vi "Test_for_6581.vi"() -> ()   [LabVIEW 2018]
uses:
  <vilib>/Platform/TimedLoop/XDataNode/timing_clust.ctl
  <vilib>/Platform/TimedLoop/XDataNode/nitl_modes.ctl
  <vilib>/Platform/TimedLoop/XDataNode/wakeup.ctl
  <vilib>/rvi/eio/common/nirviEmuTemplateMethod_errors.vi
  <vilib>/rvi/Emulation/niFpgaSctlEmulationGetInTimedLoop.vi
  <vilib>/rvi/Emulation/niFpgaEmulationReportErrorSimple.vi
  <vilib>/rvi/Emulation/niFpgaGetClockAttributes.vi
  <vilib>/rvi/Emulation/niFpgaCriticalErrorInLSC.vi
  <vilib>/eio/EIONode/EIONode.xnode
  <vilib>/Platform/TimedLoop/XDataNode/XDataNode.xnode
  <vilib>/Platform/TimedLoop/XDataNode/XDNodeRunTimeDep.lvlib
panel:
  in  "Internal Power Supply Voltage":u8(ring) items=["3.3 Volts", "2.5 Volts", "1.8 Volts"]
  in  "Supply Select":u8(ring) items=["Local", "External"]
  in  "Devider Frequency 160/(x*2), x>0":u8=1 min=1
  in  "Constant(F) / Frequency(T)":bool
  in  "IO Module\\DDCB_PFI3_Write":bool
  in  "IO Module\\DDCB_PFI2_Write":bool
  in  "IO Module\\DDCB_PFI1_Write":bool
  in  "IO Module\\DDCB_DIO23_Write":bool
  in  "IO Module\\DDCB_DIO22_Write":bool
  in  "IO Module\\DDCB_DIO21_Write":bool
  in  "IO Module\\DDCB_DIO20_Write":bool
  in  "IO Module\\DDCB_DIO19_Write":bool
  in  "IO Module\\DDCB_DIO18_Write":bool
  in  "IO Module\\DDCB_DIO17_Write":bool
  in  "IO Module\\DDCB_DIO16_Write":bool
  in  "IO Module\\DDCB_DIO15_Write":bool
  in  "IO Module\\DDCB_DIO14_Write":bool
  in  "IO Module\\DDCB_DIO13_Write":bool
  in  "IO Module\\DDCB_DIO12_Write":bool
  in  "IO Module\\DDCB_DIO11_Write":bool
  in  "IO Module\\DDCB_DIO10_Write":bool
  in  "IO Module\\DDCB_DIO9_Write":bool
  in  "IO Module\\DDCB_DIO8_Write":bool
  in  "IO Module\\DDCB_DIO7_Write":bool
  in  "IO Module\\DDCB_DIO6_Write":bool
  in  "IO Module\\DDCB_DIO5_Write":bool
  in  "IO Module\\DDCB_DIO4_Write":bool
  in  "IO Module\\DDCB_DIO3_Write":bool
  in  "IO Module\\DDCB_DIO2_Write":bool
  in  "IO Module\\DDCB_DIO1_Write":bool
  in  "IO Module\\DDCB_DIO0_Write":bool
  in  "IO Module\\DDCA_PFI3_Write":bool
  in  "IO Module\\DDCA_PFI2_Write":bool
  in  "IO Module\\DDCA_PFI1_Write":bool
  in  "IO Module\\DDCA_DIO23_Write":bool
  in  "IO Module\\DDCA_DIO22_Write":bool
  in  "IO Module\\DDCA_DIO21_Write":bool
  in  "IO Module\\DDCA_DIO20_Write":bool
  in  "IO Module\\DDCA_DIO19_Write":bool
  in  "IO Module\\DDCA_DIO18_Write":bool
  in  "IO Module\\DDCA_DIO17_Write":bool
  in  "IO Module\\DDCA_DIO16_Write":bool
  in  "IO Module\\DDCA_DIO15_Write":bool
  in  "IO Module\\DDCA_DIO14_Write":bool
  in  "IO Module\\DDCA_DIO13_Write":bool
  in  "IO Module\\DDCA_DIO12_Write":bool
  in  "IO Module\\DDCA_DIO11_Write":bool
  in  "IO Module\\DDCA_DIO10_Write":bool
  in  "IO Module\\DDCA_DIO9_Write":bool
  in  "IO Module\\DDCA_DIO8_Write":bool
  in  "IO Module\\DDCA_DIO7_Write":bool
  in  "IO Module\\DDCA_DIO6_Write":bool
  in  "IO Module\\DDCA_DIO5_Write":bool
  in  "IO Module\\DDCA_DIO4_Write":bool
  in  "IO Module\\DDCA_DIO3_Write":bool
  in  "IO Module\\DDCA_DIO2_Write":bool
  in  "IO Module\\DDCA_DIO1_Write":bool
  in  "IO Module\\DDCA_DIO0_Write":bool
  in  "Стоп":bool
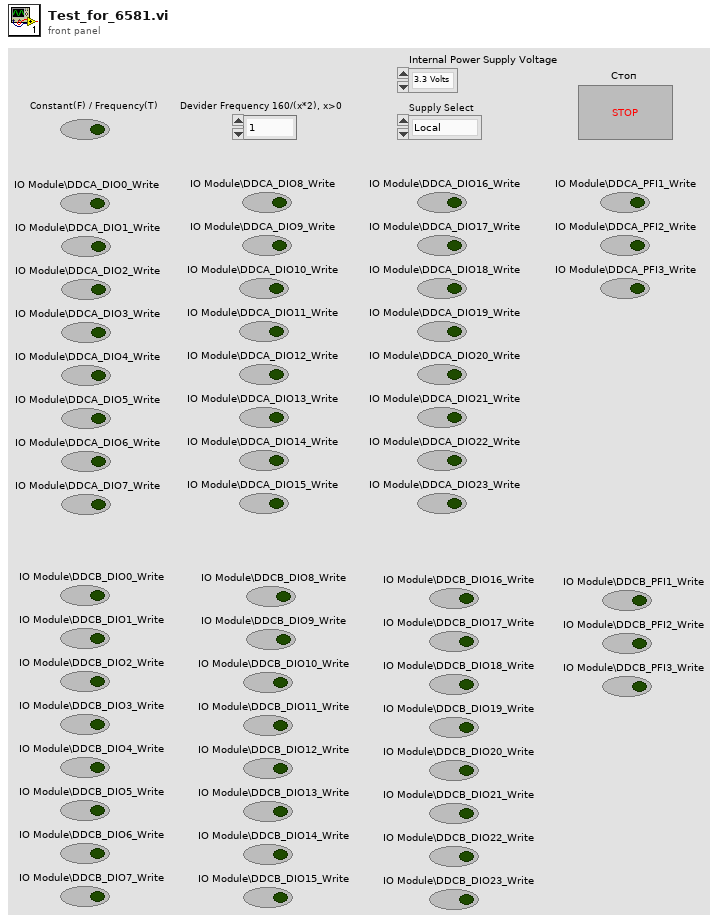
[diagram p1: front panel]
types:
  T1 = typedef "XDNodeRunTimeDep.lvlib/timing_clust.ctl" = cluster{"Expected End [f-1]":u64, "Actual End [f-1]":u64, "Finished Late? [f-1]":bool, "Expected End [i-1]":u64, "Actual End [i-1]":u64, "Finished Late? [i-1]":bool, "Expected Start [i]":u64, "Actual Start [i]":u64, "Expected Start [f]":u64, "Actual Start [f]":u64, "Source Name":string, "Structure Name":string, "Period":i64, "Deadline":i64, "Offset":i64, "Start":i64, "Priority":i32, "Timeout":i32, "Mode":T2, "Wakeup Reason":T3, "Error":errorcluster, "Source Type":string, "Secondary Source Type":string, "Global End Time":u64, "Global Start Time":u64, "Frame Duration":u64, "Iteration Duration":u64, "Assigned CPU":i32, "I/O Scan Engine Mode":u32}
  T2 = typedef "XDNodeRunTimeDep.lvlib/nitl_modes.ctl" = enum32{"No Change", "Process missed periods, maintain original phase", "Discard missed periods, maintain original phase", "Process missed periods, ignore original phase", "Discard missed periods, ignore original phase"}
  T3 = typedef "XDNodeRunTimeDep.lvlib/wakeup.ctl" = enum32{"Normal", "Aborted", "Asynchronous wakeup", "Timing source error", "Timed loop error", "Timeout"}
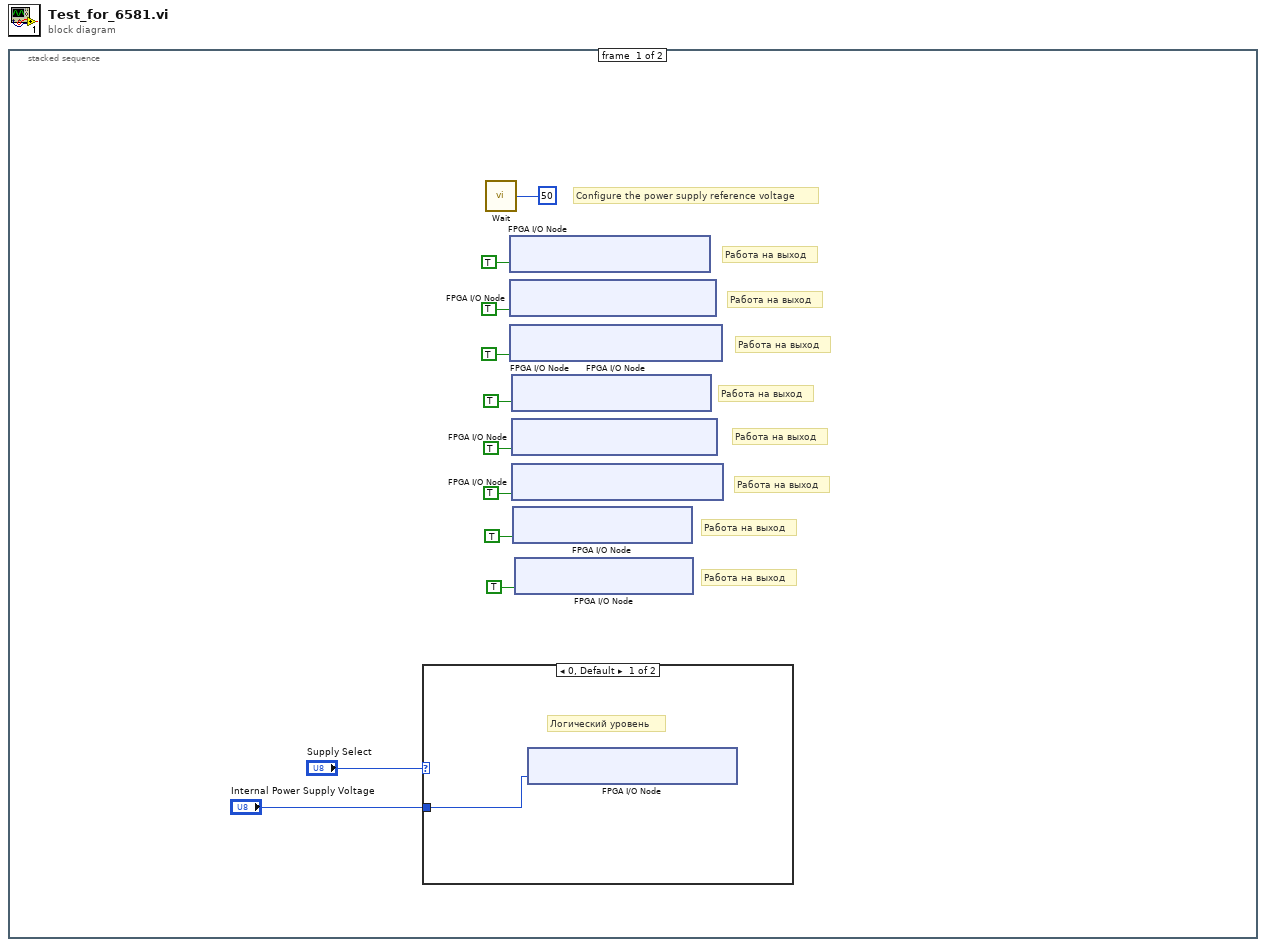
[diagram p0: block diagram]
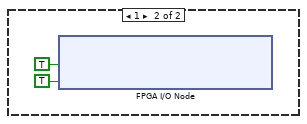
[diagram p2: hidden frame]
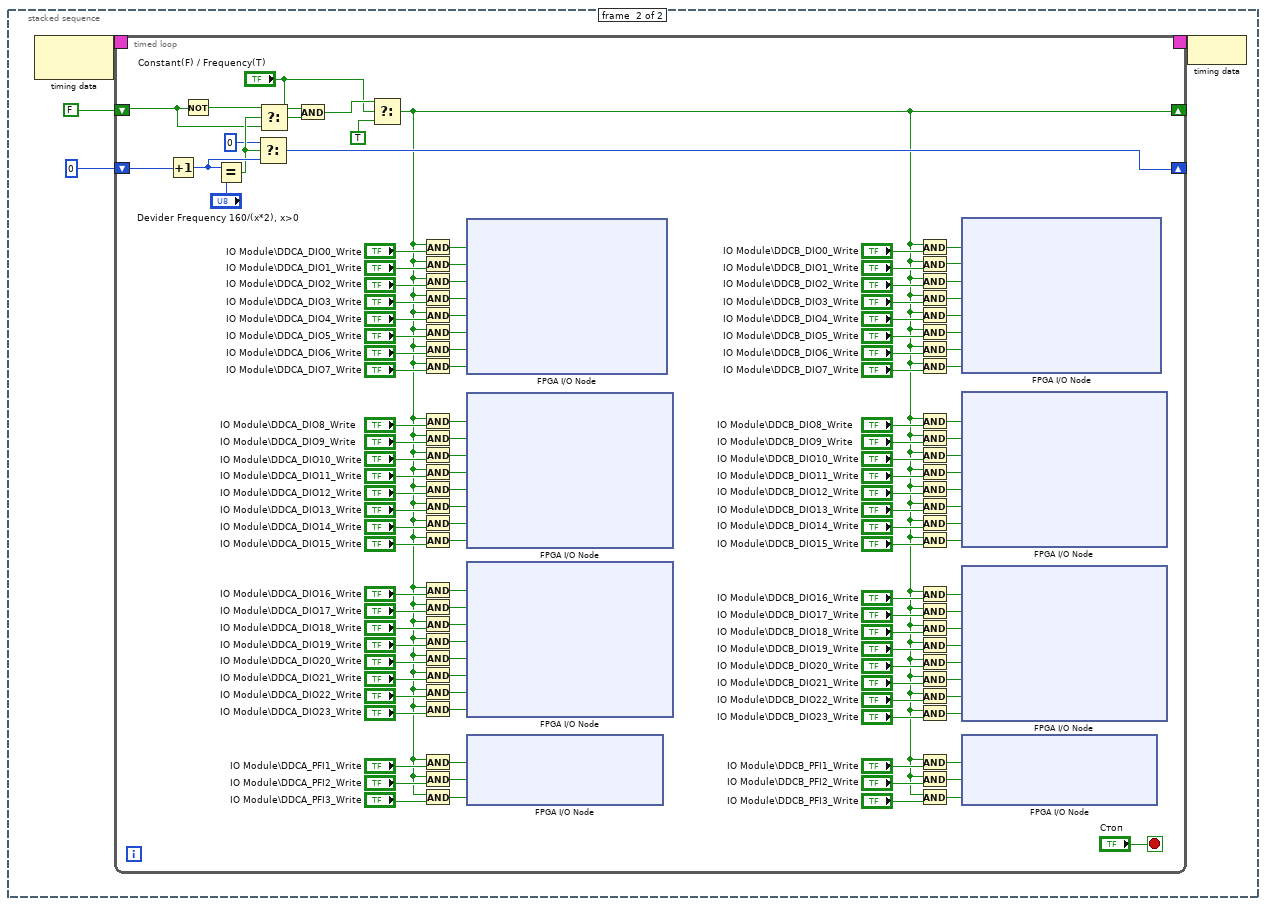
[diagram p3: hidden frame]
diagram:
  n1 = stacked-sequence {
    frame #0 {
      # "Configure the power supply reference voltage"
      # "Работа на выход"
      # "Работа на выход"
      # "Работа на выход"
      # "Работа на выход"
      # "Работа на выход"
      # "Работа на выход"
      # "Работа на выход"
      # "Работа на выход"
      n2 = case shown="0, Default" "Supply Select" {
        tunnel: "Internal Power Supply Voltage" -> [w12 _]
        frame 0, Default {
          # "Логический уровень"
          n3 = xnode "FPGA I/O Node"("IO Module\\Local_Supply_Select"=w12) -> ()  [unwired: 1 in, 1 out]
        }
        frame 1 {
          n4 = xnode "FPGA I/O Node"("IO Module\\DDCA_Supply_Select"=TRUE ("IO Module\\DDCA_Supply_Select"), "IO Module\\DDCB_Supply_Select"=TRUE ("IO Module\\DDCB_Supply_Select")) -> ()  [unwired: 2 in, 2 out]
        }
      }
      n5 = call "Wait"("Count(mSec)"=u8 50) -> ()  [unwired: 1 out]
      n6 = xnode "FPGA I/O Node"("IO Module\\DDCA_DIO0-7_WE"=TRUE ("IO Module\\DDCA_DIO0-7_WE")) -> ()  [unwired: 1 in, 1 out]
      n7 = xnode "FPGA I/O Node"("IO Module\\DDCA_DIO8-15_WE"=TRUE ("IO Module\\DDCA_DIO8-15_WE")) -> ()  [unwired: 1 in, 1 out]
      n8 = xnode "FPGA I/O Node"("IO Module\\DDCA_DIO16-23_WE"=TRUE ("IO Module\\DDCA_DIO8-15_WE")) -> ()  [unwired: 1 in, 1 out]
      n9 = xnode "FPGA I/O Node"("IO Module\\DDCB_DIO0-7_WE"=TRUE ("IO Module\\DDCA_DIO0-7_WE")) -> ()  [unwired: 1 in, 1 out]
      n10 = xnode "FPGA I/O Node"("IO Module\\DDCB_DIO8-15_WE"=TRUE ("IO Module\\DDCA_DIO8-15_WE")) -> ()  [unwired: 1 in, 1 out]
      n11 = xnode "FPGA I/O Node"("IO Module\\DDCB_DIO16-23_WE"=TRUE ("IO Module\\DDCA_DIO8-15_WE")) -> ()  [unwired: 1 in, 1 out]
      n12 = xnode "FPGA I/O Node"("IO Module\\DDCA_PFI_WE"=TRUE ("IO Module\\DDCA_DIO8-15_WE")) -> ()  [unwired: 1 in, 1 out]
      n13 = xnode "FPGA I/O Node"("IO Module\\DDCB_PFI_WE"=TRUE ("IO Module\\DDCA_DIO8-15_WE")) -> ()  [unwired: 1 in, 1 out]
    }
    frame #1 {
      n14 = node-c288() -> (w18:T1)  [unwired: 1 in]
      n15 = timed-loop {
        timing: w18 -> [_]
        timing-out: [_] -> w17
        shift-right: [w38] -> _
        shift-left: FALSE -> [w133]
        shift-right: [w77] -> _
        shift-left: u8 0 -> [w132]
        stop <- "Стоп" stop-if-true
        n16 = Increment(x=w132) -> (x+1=w137:u8)
        n17 = Not(x=w133) -> (.not. x?=w139:bool)
        n18 = Equal?(x=w137, y="Devider Frequency 160/(x*2), x>0") -> (x = y?=w136:bool)
        n19 = Select(t=u8 0, s=w136, f=w137) -> (s? t:f=w77:u8)
        n20 = Select(t=w139, s=w136, f=w133) -> (s? t:f=w134:bool)
        n21 = And(x="Constant(F) / Frequency(T)", y=w134) -> (x .and. y?=w21:bool)
        n22 = Select(t=w21, s="Constant(F) / Frequency(T)", f=TRUE ("t")) -> (s? t:f=w38:bool)
        n23 = And(x=w38, y="IO Module\\DDCA_DIO0_Write") -> (x .and. y?=w131:bool)
        n24 = And(x=w38, y="IO Module\\DDCA_DIO1_Write") -> (x .and. y?=w129:bool)
        n25 = And(x=w38, y="IO Module\\DDCA_DIO2_Write") -> (x .and. y?=w130:bool)
        n26 = And(x=w38, y="IO Module\\DDCA_DIO3_Write") -> (x .and. y?=w124:bool)
        n27 = And(x=w38, y="IO Module\\DDCA_DIO4_Write") -> (x .and. y?=w125:bool)
        n28 = And(x=w38, y="IO Module\\DDCA_DIO5_Write") -> (x .and. y?=w126:bool)
        n29 = And(x=w38, y="IO Module\\DDCA_DIO6_Write") -> (x .and. y?=w127:bool)
        n30 = And(x=w38, y="IO Module\\DDCA_DIO7_Write") -> (x .and. y?=w128:bool)
        n31 = And(x=w38, y="IO Module\\DDCA_DIO8_Write") -> (x .and. y?=w115:bool)
        n32 = And(x=w38, y="IO Module\\DDCA_DIO9_Write") -> (x .and. y?=w114:bool)
        n33 = And(x=w38, y="IO Module\\DDCA_DIO10_Write") -> (x .and. y?=w108:bool)
        n34 = And(x=w38, y="IO Module\\DDCA_DIO11_Write") -> (x .and. y?=w109:bool)
        n35 = And(x=w38, y="IO Module\\DDCA_DIO12_Write") -> (x .and. y?=w110:bool)
        n36 = And(x=w38, y="IO Module\\DDCA_DIO13_Write") -> (x .and. y?=w111:bool)
        n37 = And(x=w38, y="IO Module\\DDCA_DIO14_Write") -> (x .and. y?=w112:bool)
        n38 = And(x=w38, y="IO Module\\DDCA_DIO15_Write") -> (x .and. y?=w113:bool)
        n39 = And(x=w38, y="IO Module\\DDCA_DIO16_Write") -> (x .and. y?=w97:bool)
        n40 = And(x=w38, y="IO Module\\DDCA_DIO17_Write") -> (x .and. y?=w96:bool)
        n41 = And(x=w38, y="IO Module\\DDCA_DIO18_Write") -> (x .and. y?=w95:bool)
        n42 = And(x=w38, y="IO Module\\DDCA_DIO19_Write") -> (x .and. y?=w94:bool)
        n43 = And(x=w38, y="IO Module\\DDCA_DIO20_Write") -> (x .and. y?=w93:bool)
        n44 = And(x=w38, y="IO Module\\DDCA_DIO21_Write") -> (x .and. y?=w92:bool)
        n45 = And(x=w38, y="IO Module\\DDCA_DIO22_Write") -> (x .and. y?=w98:bool)
        n46 = And(x=w38, y="IO Module\\DDCA_DIO23_Write") -> (x .and. y?=w99:bool)
        n47 = And(x=w38, y="IO Module\\DDCA_PFI1_Write") -> (x .and. y?=w81:bool)
        n48 = And(x=w38, y="IO Module\\DDCA_PFI2_Write") -> (x .and. y?=w82:bool)
        n49 = And(x=w38, y="IO Module\\DDCA_PFI3_Write") -> (x .and. y?=w83:bool)
        n50 = xnode "FPGA I/O Node"("IO Module\\DDCA_DIO0_Write"=w131, "IO Module\\DDCA_DIO1_Write"=w129, "IO Module\\DDCA_DIO2_Write"=w130, "IO Module\\DDCA_DIO3_Write"=w124, "IO Module\\DDCA_DIO4_Write"=w125, "IO Module\\DDCA_DIO5_Write"=w126, "IO Module\\DDCA_DIO6_Write"=w127, "IO Module\\DDCA_DIO7_Write"=w128) -> ()  [unwired: 8 in, 8 out]
        n51 = xnode "FPGA I/O Node"("IO Module\\DDCA_DIO8_Write"=w115, "IO Module\\DDCA_DIO9_Write"=w114, "IO Module\\DDCA_DIO10_Write"=w108, "IO Module\\DDCA_DIO11_Write"=w109, "IO Module\\DDCA_DIO12_Write"=w110, "IO Module\\DDCA_DIO13_Write"=w111, "IO Module\\DDCA_DIO14_Write"=w112, "IO Module\\DDCA_DIO15_Write"=w113) -> ()  [unwired: 8 in, 8 out]
        n52 = xnode "FPGA I/O Node"("IO Module\\DDCA_DIO16_Write"=w97, "IO Module\\DDCA_DIO17_Write"=w96, "IO Module\\DDCA_DIO18_Write"=w95, "IO Module\\DDCA_DIO19_Write"=w94, "IO Module\\DDCA_DIO20_Write"=w93, "IO Module\\DDCA_DIO21_Write"=w92, "IO Module\\DDCA_DIO22_Write"=w98, "IO Module\\DDCA_DIO23_Write"=w99) -> ()  [unwired: 8 in, 8 out]
        n53 = xnode "FPGA I/O Node"("IO Module\\DDCA_PFI1_Write"=w81, "IO Module\\DDCA_PFI2_Write"=w82, "IO Module\\DDCA_PFI3_Write"=w83) -> ()  [unwired: 3 in, 3 out]
        n54 = And(x=w38, y="IO Module\\DDCB_DIO0_Write") -> (x .and. y?=w37:bool)
        n55 = And(x=w38, y="IO Module\\DDCB_DIO1_Write") -> (x .and. y?=w36:bool)
        n56 = And(x=w38, y="IO Module\\DDCB_DIO2_Write") -> (x .and. y?=w35:bool)
        n57 = And(x=w38, y="IO Module\\DDCB_DIO3_Write") -> (x .and. y?=w34:bool)
        n58 = And(x=w38, y="IO Module\\DDCB_DIO4_Write") -> (x .and. y?=w33:bool)
        n59 = And(x=w38, y="IO Module\\DDCB_DIO5_Write") -> (x .and. y?=w32:bool)
        n60 = And(x=w38, y="IO Module\\DDCB_DIO6_Write") -> (x .and. y?=w31:bool)
        n61 = And(x=w38, y="IO Module\\DDCB_DIO7_Write") -> (x .and. y?=w30:bool)
        n62 = And(x=w38, y="IO Module\\DDCB_DIO8_Write") -> (x .and. y?=w29:bool)
        n63 = And(x=w38, y="IO Module\\DDCB_DIO9_Write") -> (x .and. y?=w28:bool)
        n64 = And(x=w38, y="IO Module\\DDCB_DIO10_Write") -> (x .and. y?=w27:bool)
        n65 = And(x=w38, y="IO Module\\DDCB_DIO11_Write") -> (x .and. y?=w26:bool)
        n66 = And(x=w38, y="IO Module\\DDCB_DIO12_Write") -> (x .and. y?=w25:bool)
        n67 = And(x=w38, y="IO Module\\DDCB_DIO13_Write") -> (x .and. y?=w24:bool)
        n68 = And(x=w38, y="IO Module\\DDCB_DIO14_Write") -> (x .and. y?=w23:bool)
        n69 = And(x=w38, y="IO Module\\DDCB_DIO15_Write") -> (x .and. y?=w22:bool)
        n70 = And(x=w38, y="IO Module\\DDCB_DIO16_Write") -> (x .and. y?=w66:bool)
        n71 = And(x=w38, y="IO Module\\DDCB_DIO17_Write") -> (x .and. y?=w67:bool)
        n72 = And(x=w38, y="IO Module\\DDCB_DIO18_Write") -> (x .and. y?=w68:bool)
        n73 = And(x=w38, y="IO Module\\DDCB_DIO19_Write") -> (x .and. y?=w69:bool)
        n74 = And(x=w38, y="IO Module\\DDCB_DIO20_Write") -> (x .and. y?=w70:bool)
        n75 = And(x=w38, y="IO Module\\DDCB_DIO21_Write") -> (x .and. y?=w71:bool)
        n76 = And(x=w38, y="IO Module\\DDCB_DIO22_Write") -> (x .and. y?=w72:bool)
        n77 = And(x=w38, y="IO Module\\DDCB_DIO23_Write") -> (x .and. y?=w73:bool)
        n78 = And(x=w38, y="IO Module\\DDCB_PFI1_Write") -> (x .and. y?=w74:bool)
        n79 = And(x=w38, y="IO Module\\DDCB_PFI2_Write") -> (x .and. y?=w75:bool)
        n80 = And(x=w38, y="IO Module\\DDCB_PFI3_Write") -> (x .and. y?=w76:bool)
        n81 = xnode "FPGA I/O Node"("IO Module\\DDCB_DIO0_Write"=w37, "IO Module\\DDCB_DIO1_Write"=w36, "IO Module\\DDCB_DIO2_Write"=w35, "IO Module\\DDCB_DIO3_Write"=w34, "IO Module\\DDCB_DIO4_Write"=w33, "IO Module\\DDCB_DIO5_Write"=w32, "IO Module\\DDCB_DIO6_Write"=w31, "IO Module\\DDCB_DIO7_Write"=w30) -> ()  [unwired: 8 in, 8 out]
        n82 = xnode "FPGA I/O Node"("IO Module\\DDCB_DIO8_Write"=w29, "IO Module\\DDCB_DIO9_Write"=w28, "IO Module\\DDCB_DIO10_Write"=w27, "IO Module\\DDCB_DIO11_Write"=w26, "IO Module\\DDCB_DIO12_Write"=w25, "IO Module\\DDCB_DIO13_Write"=w24, "IO Module\\DDCB_DIO14_Write"=w23, "IO Module\\DDCB_DIO15_Write"=w22) -> ()  [unwired: 8 in, 8 out]
        n83 = xnode "FPGA I/O Node"("IO Module\\DDCB_DIO16_Write"=w66, "IO Module\\DDCB_DIO17_Write"=w67, "IO Module\\DDCB_DIO18_Write"=w68, "IO Module\\DDCB_DIO19_Write"=w69, "IO Module\\DDCB_DIO20_Write"=w70, "IO Module\\DDCB_DIO21_Write"=w71, "IO Module\\DDCB_DIO22_Write"=w72, "IO Module\\DDCB_DIO23_Write"=w73) -> ()  [unwired: 8 in, 8 out]
        n84 = xnode "FPGA I/O Node"("IO Module\\DDCB_PFI1_Write"=w74, "IO Module\\DDCB_PFI2_Write"=w75, "IO Module\\DDCB_PFI3_Write"=w76) -> ()  [unwired: 3 in, 3 out]
      }
      n85 = node-c288(w17) -> ()
    }
  }
